vi "readLidar.vi"(5 "robotPos":cluster{"xPos":dbl, "yPos":dbl, "theta":dbl}, 6 "error in":errorcluster, 8 "VISA resource name in":refnum<visa-resource-name>) -> (0 "error out":errorcluster, 1 "stop":bool, 2 "VISA resource name out":refnum<visa-resource-name>, 3 "line out":cluster{"Line":cluster{"X":dbl, "Y":dbl}[]}[](array[cluster]))   [LabVIEW 2016]
uses:
  <instrlib>/Hokuyo URG Series/Hokuyo URG Series.lvlib
panel:
  in  "upsideDown?":bool=TRUE
  out "XY Graph 1.5m max":cluster{"Line":cluster{"X":dbl, "Y":dbl}[]}[](graph)
  out "XY Graph 6m max":cluster{"Line":cluster{"X":dbl, "Y":dbl}[]}[](graph)
  in  "End Point":dbl=120.0
  in  "Start Point":dbl=-120.0
  in  "Cluster Count":dbl=1.0
  in  "Encoding Width":u16(ring)=3 items=["2 Byte"=2, "3 Byte"=3]
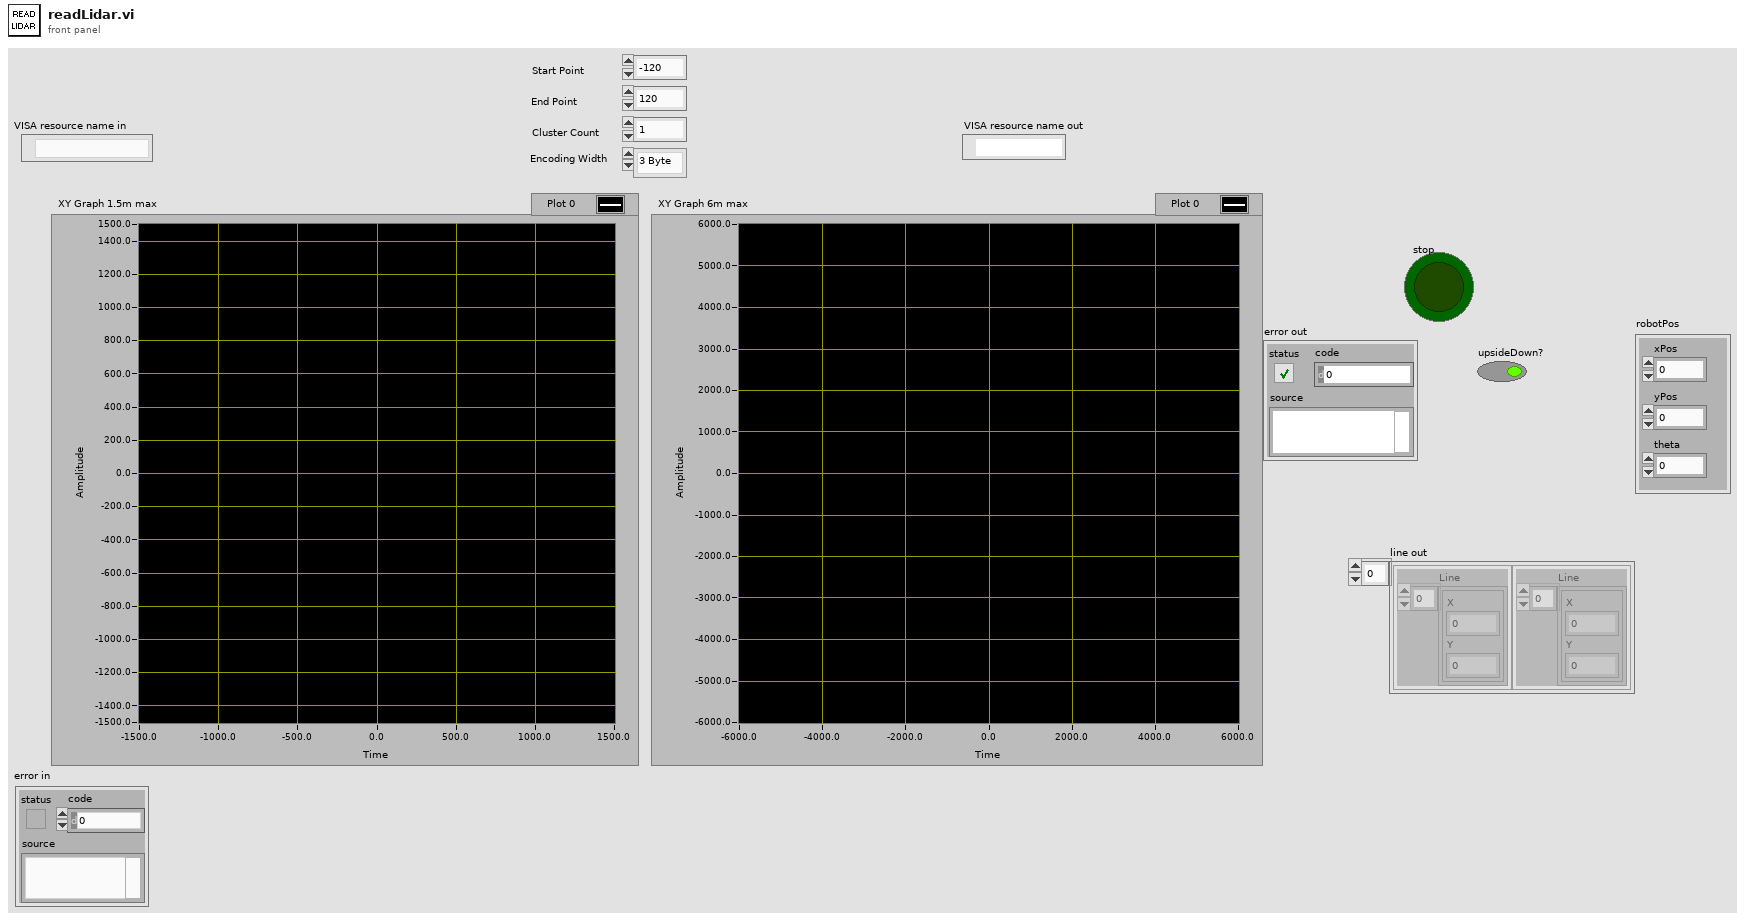
[diagram p1: front panel]
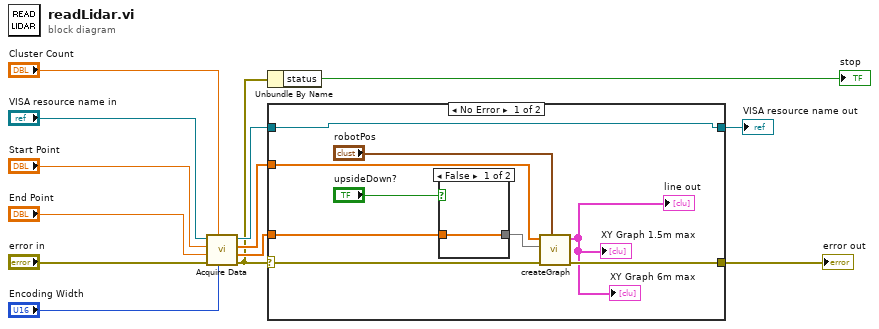
[diagram p0: block diagram]
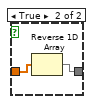
[diagram p2: hidden frame]
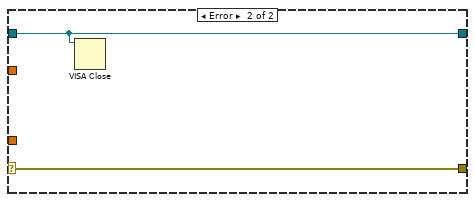
[diagram p3: hidden frame]
diagram:
  n1 = call <instrlib>:"Acquire Data.vi"("Data Encoding Width (3 Byte)"="Encoding Width", "Cluster Count (1)"="Cluster Count", "error in (no error)"="error in", "End Point (120°)"="End Point", "Start Point (-120°)"="Start Point", "VISA resource name"="VISA resource name in") -> ("error out"=w6:errorcluster, "Direction"=w7:dbl[], "Magnitude"=w8:dbl[], "VISA resource name out"=w9:refnum<visa-resource-name>)  [unwired: 2 in]
  n2 = Unbundle By Name(w6) -> ("status"=→"stop":bool)
  n3 = case shown="No Error" w6 {
    selector: w6 -> [w20 w27]
    tunnel: [w19 w27] -> w11
    tunnel: w9 -> [w22 w26]
    tunnel: [w22 w26] -> w10
    tunnel: w8 -> [w21 _]
    tunnel: w7 -> [w16 _]
    frame No Error {
      n4 = case shown="False" "upsideDown?" {
        tunnel: w16 -> [w23 w25]
        tunnel: [w23 w24] -> w15
        frame False {
        }
        frame True {
          n5 = Reverse 1D Array(array=w25) -> (reversed array=w24:dbl[])
        }
      }
      n6 = call "createGraph.vi"("robotPos"="robotPos", "error in"=w20, "Direction"=w15, "Magnitude"=w21) -> ("error out"=w19:errorcluster, "line out"=→"XY Graph 1.5m max" →"XY Graph 6m max" →"line out":cluster{"Line":cluster{"X":dbl, "Y":dbl}[]}[])  [unwired: 6 in]
    }
    frame Error {
      n7 = VISA Close(VISA resource name=w26) -> ()  [unwired: 1 in, 1 out]
    }
  }
  "error out" <- w11
  "VISA resource name out" <- w10
